vi "BallDispPosSkillVSS.vi"(8 "error in (no error)":errorcluster, 9 "Game":refnum<class "Game.lvclass">, 10 "Robot in":refnum<class "Robot.lvclass">, 11 "BallDispPosSkillVSS in":refnum<class "BallDispPosSkillVSS.lvclass">) -> (0 "error out":errorcluster, 2 "Robot out":refnum<class "Robot.lvclass">, 3 "BallDispPosSkillVSS out":refnum<class "BallDispPosSkillVSS.lvclass">)   [LabVIEW 2023, in "BallDispPosSkillVSS.lvclass"]
uses:
  BallDispPosSkillVSS.lvclass
  Robot_class/Robot.lvclass
  Game_class/Game.lvclass
  Game_class/Game.lvclass/Game.ctl
  Object_class/Object.lvclass/Object.ctl
  Robot_class/Robot.lvclass/Robot.ctl
  Game_class/Read BallRef.vi
  Object_class/Read y.vi
  Object_class/Read x.vi
  Robot_class/Write dest_y.vi
  Robot_class/Write dest_x.vi
  Robot_class/Write dest_orientation.vi
  Ball_class/Ball.lvclass
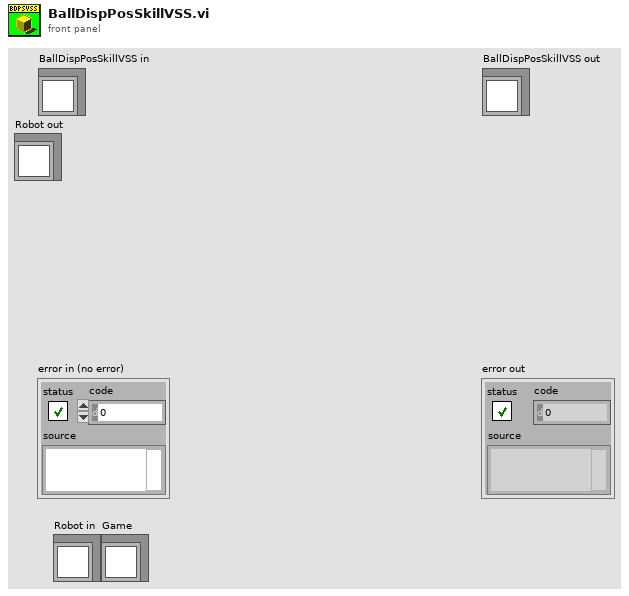
[diagram p1: front panel]
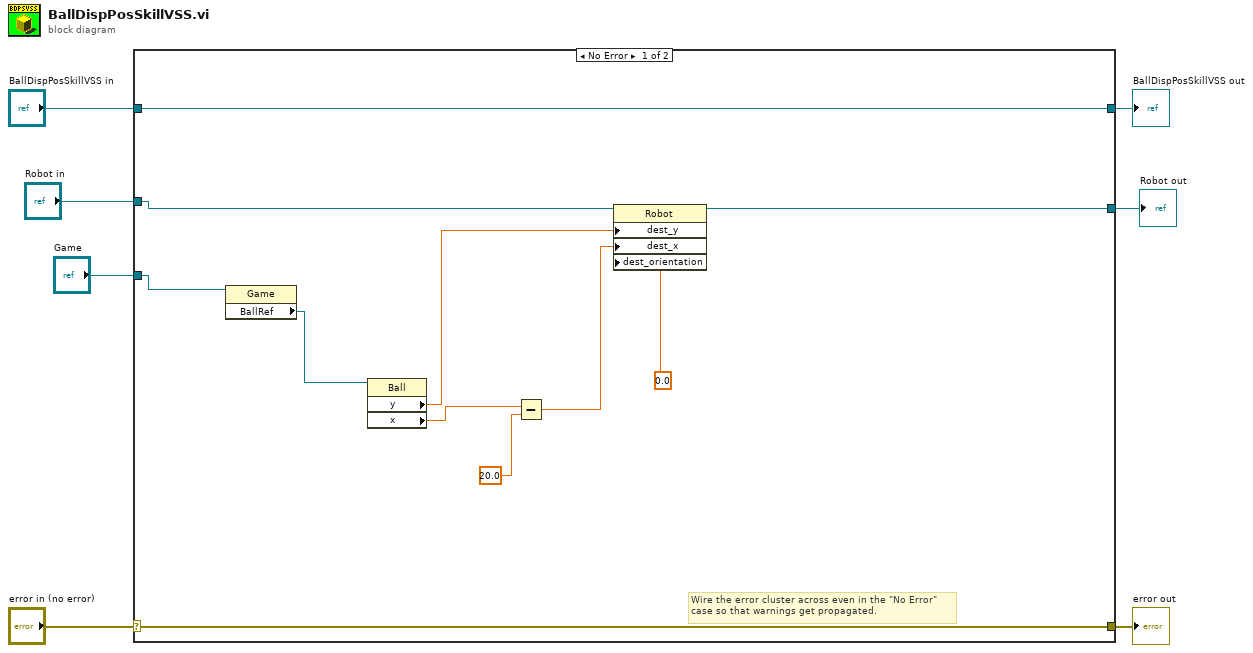
[diagram p0: block diagram]
diagram:
  n1 = case shown="No Error" "error in (no error)" {
    selector: "error in (no error)" -> [w17 w21]
    tunnel: [w17 w21] -> w6
    tunnel: [w18 w20] -> w4
    tunnel: "BallDispPosSkillVSS in" -> [w18 w20]
    tunnel: "Robot in" -> [w9 w19]
    tunnel: "Game" -> [w11 _]
    tunnel: [w8 w19] -> w1
    frame No Error {
      # "Wire the error cluster across even in the \"No Error\"\ncase so that warnings get propagated."
      n2 = property class="Game"(reference=w11) -> ("BallRef"=w10:refnum<class "Ball.lvclass">)  [unwired: 1 in, 2 out]
      n3 = property class="Ball"(reference=w10) -> ("y"=w12:dbl, "x"=w14:dbl)  [unwired: 1 in, 2 out]
      n4 = Subtract(x=w14, y=20.0) -> (x-y=w13:dbl)
      n5 = property class="Robot"(reference=w9, "dest_y"=w12, "dest_x"=w13, "dest_orientation"=0.0) -> (reference out=w8:refnum<class "Robot.lvclass">)  [unwired: 1 in, 1 out]
    }
    frame Error {
    }
  }
  "error out" <- w6
  "BallDispPosSkillVSS out" <- w4
  "Robot out" <- w1
